vi "ATSh_InputControl.vi"(6 "Impedance":u32, 8 "InputRange":u32, 9 "Coupling":u32, 10 "Channel":u32, 11 "HandleIn":u32) -> (0 "Return":u32, 2 "Channel_Out":u32, 3 "Handle_Out":u32)   [LabVIEW 2015]
doc: "_____AlazarTech, Scope_____\n\nConfigure an input channel circuitry.\nHandle input.\n\nChannel:\n - A : 0x01\n - B : 0x02\n\nCoupling:\n - AC : 0x01\n - DC : 0x02\n\nInputRange:\n - 20_MV 0x001\n - 40_MV 0x002\n - 50_MV 0x003\n - 80_MV 0x004\n -100_MV 0x005\n -200_MV 0x006\n -400_MV 0x007\n -500_MV 0x008\n -800_MV 0x009\n - 1_V 0x00A\n - 2_V 0x00B\n - 4_V 0x00C\n - 5_V 0x00D\n - 8_V 0x00E\n - 10_V 0x00F\n - 16_V 0x012\n - 20_V 0x010\n - 40_V 0x011\n - HiFi 0x020\n\nImpedance:\n - 1M_OHMS 0x001\n - 50_OHMS 0x002"
uses:
  ATSApi.dll
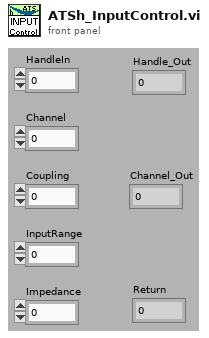
[diagram p1: front panel]
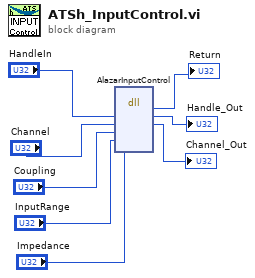
[diagram p0: block diagram]
diagram:
  n1 = dll-call lib="C:/IntensityOCT/trunk/ATSApi.dll" fn="AlazarInputControl"("h"="HandleIn", "Channel"="Channel", "Coupling"="Coupling", "InputRange"="InputRange", "Impedance"="Impedance") -> (→"Return":u32, "h"=→"Handle_Out":u32, "Channel"=→"Channel_Out":u32)  [unwired: 6 in, 2 out]
